vi "sc_getXYZPosition.vi"(0 "VISA handle 2":refnum<visa-resource-name>, 11 "error in (no error) 2":errorcluster) -> (4 "Dup. VISA handle 2":refnum<visa-resource-name>, 6 "X pos (steps)":i32, 8 "Y pos (steps)":i32, 10 "Z pos (steps)":i32, 15 "error out 2":errorcluster)   [LabVIEW 2019]
uses:
  controls/scientifica_commands.ctl
panel:
  out "Position (text)":string
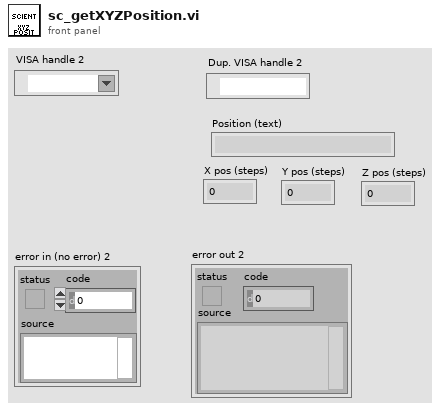
[diagram p1: front panel]
types:
  T1 = typedef "scientifica_commands.ctl" = enum16{"ANGLE", "INSET", "FIRST", "ZERO", "Pz", "P", "absz", "ACC", "TOP", "STOP", "rel", "relz", "abs", "IN", "vj", "APROACH", "OBJS", "OBJU", "OUT", "OBJ", "OBJL", "SET", "OBJD", "STEP", "SETSTEP", "S", "UUX", "UUY", "UUZ"}
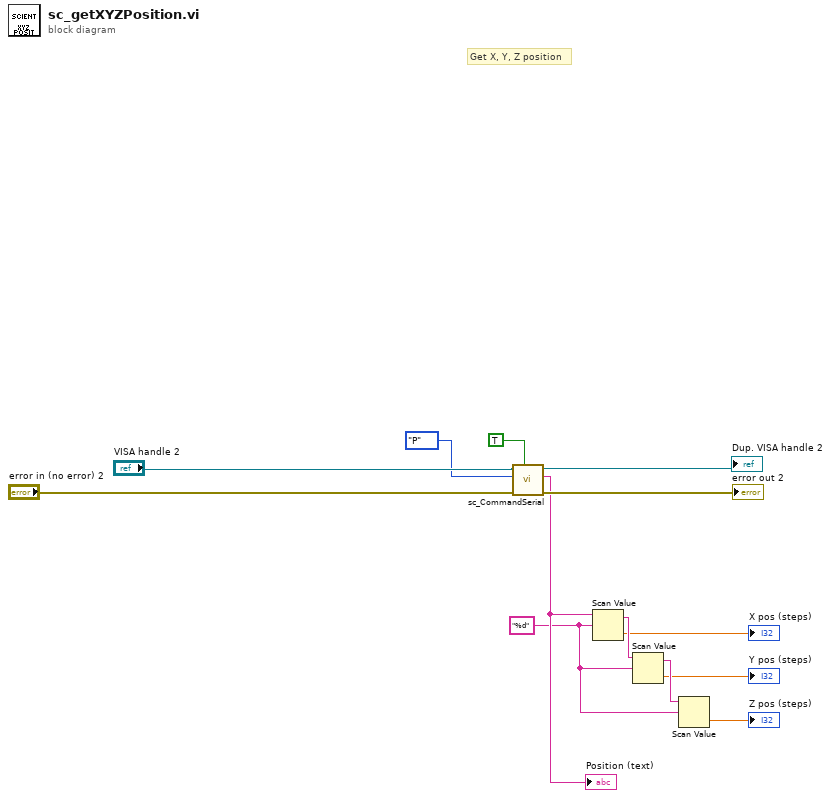
[diagram p0: block diagram]
diagram:
  w5 = "%d" ("format string")
  # "Get X, Y, Z position"
  n1 = call "sc_CommandSerial.vi"("Query?"=TRUE, "error in (no error)"="error in (no error) 2", "Scientifica commands"=scientifica_commands."P", "VISA handle"="VISA handle 2") -> ("error out"=→"error out 2":errorcluster, "Response"=w7:string, "Dup. VISA handle"=→"Dup. VISA handle 2":refnum<visa-resource-name>)  [unwired: 4 in, 1 out]
  "Position (text)" <- w7
  n2 = Scan Value(string=w7, format string=w5) -> (output string=w6:string, value=→"X pos (steps)":dbl)  [unwired: 1 in]
  n3 = Scan Value(string=w6, format string=w5) -> (output string=w4:string, value=→"Y pos (steps)":dbl)  [unwired: 1 in]
  n4 = Scan Value(string=w4, format string=w5) -> (value=→"Z pos (steps)":dbl)  [unwired: 1 in, 1 out]
